vi "setPolaritySwitch.vi"(8 "error in (no error)":errorcluster, 9 "Switch":bool, 10 "channel index":i32, 11 "FakePressureController in":refnum<class "TDK-Lambda Z Bipolar.lvclass">) -> (0 "error out":errorcluster, 3 "FakePressureController out":refnum<class "TDK-Lambda Z Bipolar.lvclass">)   [LabVIEW 2020, in "TDK-Lambda Z Bipolar.lvclass"]
uses:
  TDK-Lambda Z Bipolar.lvclass
  TDK-Lambda Z Bipolar.lvclass/TDK-Lambda Z Bipolar.ctl
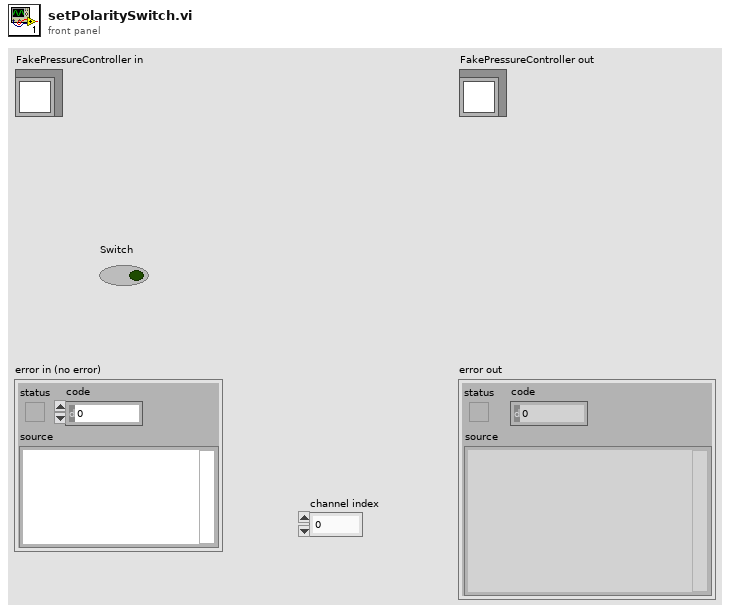
[diagram p1: front panel]
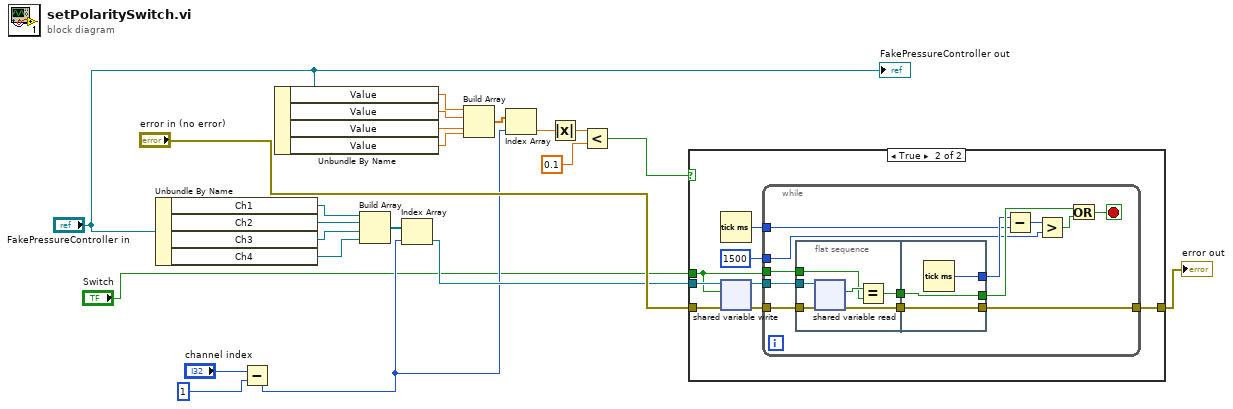
[diagram p0: block diagram]
diagram:
  n1 = Unbundle By Name("FakePressureController in") -> ("Ch1"=w19:refnum<k21>, "Ch2"=w18:refnum<k21>, "Ch3"=w17:refnum<k21>, "Ch4"=w16:refnum<k21>)
  n2 = Subtract(x="channel index", y=1) -> (x-y=w8:i32)
  n3 = Unbundle By Name("FakePressureController in") -> ("Value"=w12:dbl, "Value"=w11:dbl, "Value"=w10:dbl, "Value"=w9:dbl)
  n4 = Build Array(w19, w18, w17, w16) -> (w20:refnum<k21>[])
  n5 = Index Array(array=w20, index=w8) -> (element=w14:refnum<k21>)
  n6 = Build Array(w12, w11, w10, w9) -> (w7:dbl[])
  n7 = Index Array(array=w7, index=w8) -> (element=w6:dbl)
  n8 = Absolute Value(x=w6) -> (abs(x)=w5:dbl)
  n9 = Less?(x=w5, y=0.1) -> (x < y?=w3:bool)
  n10 = case shown="True" w3 {
    tunnel: "error in (no error)" -> [w23 w29]
    tunnel: w14 -> [_ w28]
    tunnel: [w23 w27] -> w2
    tunnel: "Switch" -> [_ w24]
    frame False {
    }
    frame True {
      n11 = Tick Count (ms)() -> (millisecond timer value=w26:u32)
      n12 = shared-variable-write(w28, w29, w24) -> (w31:refnum<k21>, w30:errorcluster)
      n13 = while {
        tunnel: w31 -> [w44]
        tunnel: w24 -> [w43]
        tunnel: w30 -> [w42]
        tunnel: [w41] -> w27
        tunnel: w26 -> [w35]
        tunnel: 1500 -> [w33]
        stop <- w37 stop-if-true
        n14 = flat-sequence {
          tunnel: w44 -> [w50]
          tunnel: w43 -> [w48]
          tunnel: w42 -> [w46]
          tunnel: [w47] -> w40
          tunnel: [w45] -> w39
          tunnel: [w52] -> w41
          tunnel: [w53] -> w38
          tunnel: w40 -> [w53]
          tunnel: w39 -> [w52]
          tunnel: [w51] -> w36
          frame #0 {
            n15 = shared-variable-read(w50, w46) -> (w45:errorcluster, w49:bool)  [unwired: 2 out]
            n16 = Equal?(x=w49, y=w48) -> (x = y?=w47:bool)
          }
          frame #1 {
            n17 = Tick Count (ms)() -> (millisecond timer value=w51:u32)
          }
        }
        n18 = Subtract(x=w36, y=w35) -> (x-y=w34:u32)
        n19 = Greater?(x=w34, y=w33) -> (0:w32:bool)
        n20 = Or(x=w38, y=w32) -> (x .or. y?=w37:bool)
      }
    }
  }
  "error out" <- w2
  "FakePressureController out" <- "FakePressureController in"
